vi "Scan1762testlongpulsetelegraph.vi"() -> ()   [LabVIEW 2012]
uses:
  <vilib>/DAQmx/write.llb/DAQmx Write (Digital Wfm 1Chan NSamp).vi
  <vilib>/DAQmx/create/channels.llb/DAQmx Create Channel (DO-Digital Output).vi
  <vilib>/DAQmx/configure/timing.llb/DAQmx Timing (Sample Clock).vi
  <vilib>/Waveform/DWDTOps.llb/DWDT Uncompress Digital.vi
  <vilib>/DAQmx/miscellaneous.llb/DAQmx Fill In Error Info.vi
  <vilib>/Utility/file.llb/Write To Spreadsheet File (DBL).vi
panel:
  out "10xwindow":i32
  out "10xdiscr":dbl
  out "DARK?":i32(graph)
  out "Counts":i32
  out "DARK?":bool
  out "PMT Counts":i32(graph)
  in  "PMT sample time":dbl=0.05
  out "Counts after 1762":i32=57
  out "OuterLoop":i32=101
  out "InnerLoop":i32=19
  out "Frequency Step Size":dbl=10000.0
  out "Bright Events":dbl
  in  "Discriminator Level\n (Bright/Dark)":i32=21
  out "number of samples written per channel\n(debug)":u32=42501
  out "digital waveform out 2":digitalwaveform(waveform)={"t0"=timestamp(0 s since 1904-01-01), "dt"=1e-07, "Y"={"transitions"=[0, 20000, 21001, 21501, 22501, 42500], "data"=[[1, 1, 0, 0], [0, 0, 0, 0], [0, 0, 0, 1], [0, 0, 0, 0], [1, 1, 0, 0], [1, 1, 0, 0]]}, "error"={"status"=FALSE, "code"=37421928, "source"=""}}
  in  "1762 pulse length (units of .1 us)":dbl=500.0
  in  "Comment":string="SPAOM, DPAOM = 77 MHz"
  in  "B Field":dbl=2.26
  in  "Power":dbl
  in  "Rerun BG Every\nnth freq point":dbl=20.0
  in  "PMT sample time":dbl=0.05
  out "Counts finding bright ion":dbl=39.0
  in  "BG Cutoff Limit":dbl=38.0
  in  "Runs per data point":dbl=20.0
  in  "Low Freq":dbl(slide)=81000000.0 min=50000000.0 max=120000000.0 step=1000.0 scale=75000000.0..90000000.0 scale format="%#.5f"
  in  "High Freq":dbl(slide)=86000000.0 min=50000000.0 max=120000000.0 step=1000.0 scale=80000000.0..90000000.0 scale format="%#.0f"
  out "Cur Freq":dbl=85984000.0 format="%#_8f"
  out "Path":path=path "c:/data/1762 Scans/2014-05-20_19-16-05_1762scanWithPumping.txt"
  out "Frequency Scan":cluster{dbl, dbl}[](graph)=[{87004000.0, 1.0}, {86994000.0, 1.0}, {86984000.0, 1.0}, {86974000.0, 1.0}, {86964000.0, 1.0}, {86954000.0, 1.0}, {86944000.0, 1.0}, {86934000.0, 1.0}, {86924000.0, 1.0}, {86914000.0, 1.0}, {86904000.0, 1.0}, {86894000.0, 1.0}, {86884000.0, 1.0}, {86874000.0, 1.0}, {86864000.0, 1.0}, {86854000.0, 1.0}, {86844000.0, 1.0}, {86834000.0, 1.0}, {86824000.0, 1.0}, {86814000.0, 1.0}, {86804000.0, 1.0}, {86794000.0, 1.0}, {86784000.0, 1.0}, {86774000.0, 1.0}, {86764000.0, 1.0}, {86754000.0, 1.0}, {86744000.0, 1.0}, {86734000.0, 1.0}, {86724000.0, 1.0}, {86714000.0, 1.0}, {86704000.0, 1.0}, {86694000.0, 1.0}, {86684000.0, 1.0}, {86674000.0, 1.0}, {86664000.0, 1.0}, {86654000.0, 1.0}, {86644000.0, 1.0}, {86634000.0, 1.0}, {86624000.0, 1.0}, {86614000.0, 1.0}, {86604000.0, 1.0}, {86594000.0, 1.0}, {86584000.0, 1.0}, {86574000.0, 1.0}, {86564000.0, 1.0}, {86554000.0, 1.0}, {86544000.0, 1.0}, {86534000.0, 1.0}, {86524000.0, 1.0}, {86514000.0, 1.0}, {86504000.0, 1.0}, {86494000.0, 1.0}, {86484000.0, 1.0}, {86474000.0, 1.0}, {86464000.0, 1.0}, {86454000.0, 1.0}, {86444000.0, 1.0}, {86434000.0, 1.0}, {86424000.0, 1.0}, {86414000.0, 1.0}, {86404000.0, 1.0}, {86394000.0, 1.0}, {86384000.0, 1.0}, {86374000.0, 1.0}, {86364000.0, 1.0}, {86354000.0, 1.0}, {86344000.0, 1.0}, {86334000.0, 1.0}, {86324000.0, 1.0}, {86314000.0, 1.0}, {86304000.0, 1.0}, {86294000.0, 1.0}, {86284000.0, 1.0}, {86274000.0, 1.0}, {86264000.0, 1.0}, {86254000.0, 1.0}, {86244000.0, 1.0}, {86234000.0, 1.0}, {86224000.0, 1.0}, {86214000.0, 1.0}, {86204000.0, 1.0}, {86194000.0, 1.0}, {86184000.0, 1.0}, {86174000.0, 1.0}, {86164000.0, 1.0}, {86154000.0, 1.0}, {86144000.0, 1.0}, {86134000.0, 1.0}, {86124000.0, 1.0}, {86114000.0, 1.0}, {86104000.0, 1.0}, {86094000.0, 1.0}, {86084000.0, 1.0}, {86074000.0, 1.0}, {86064000.0, 1.0}, {86054000.0, 1.0}, {86044000.0, 1.0}, {86034000.0, 1.0}, {86024000.0, 1.0}, {86014000.0, 1.0}, {86004000.0, 1.0}, {85994000.0, 1.0}]
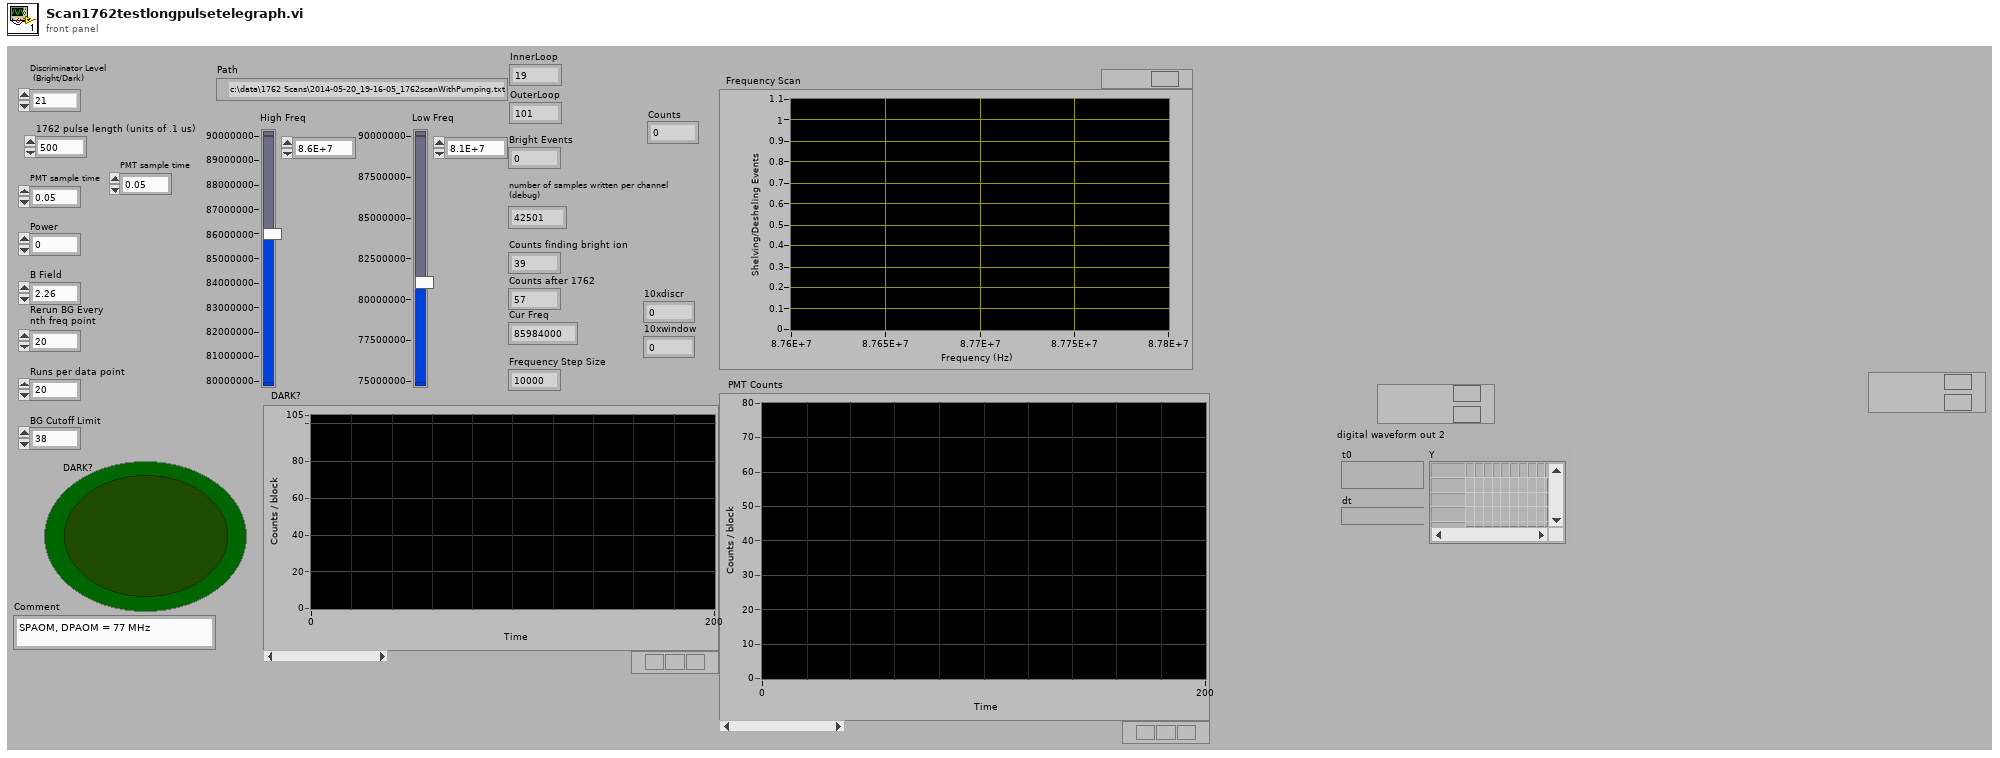
[diagram p1: front panel]
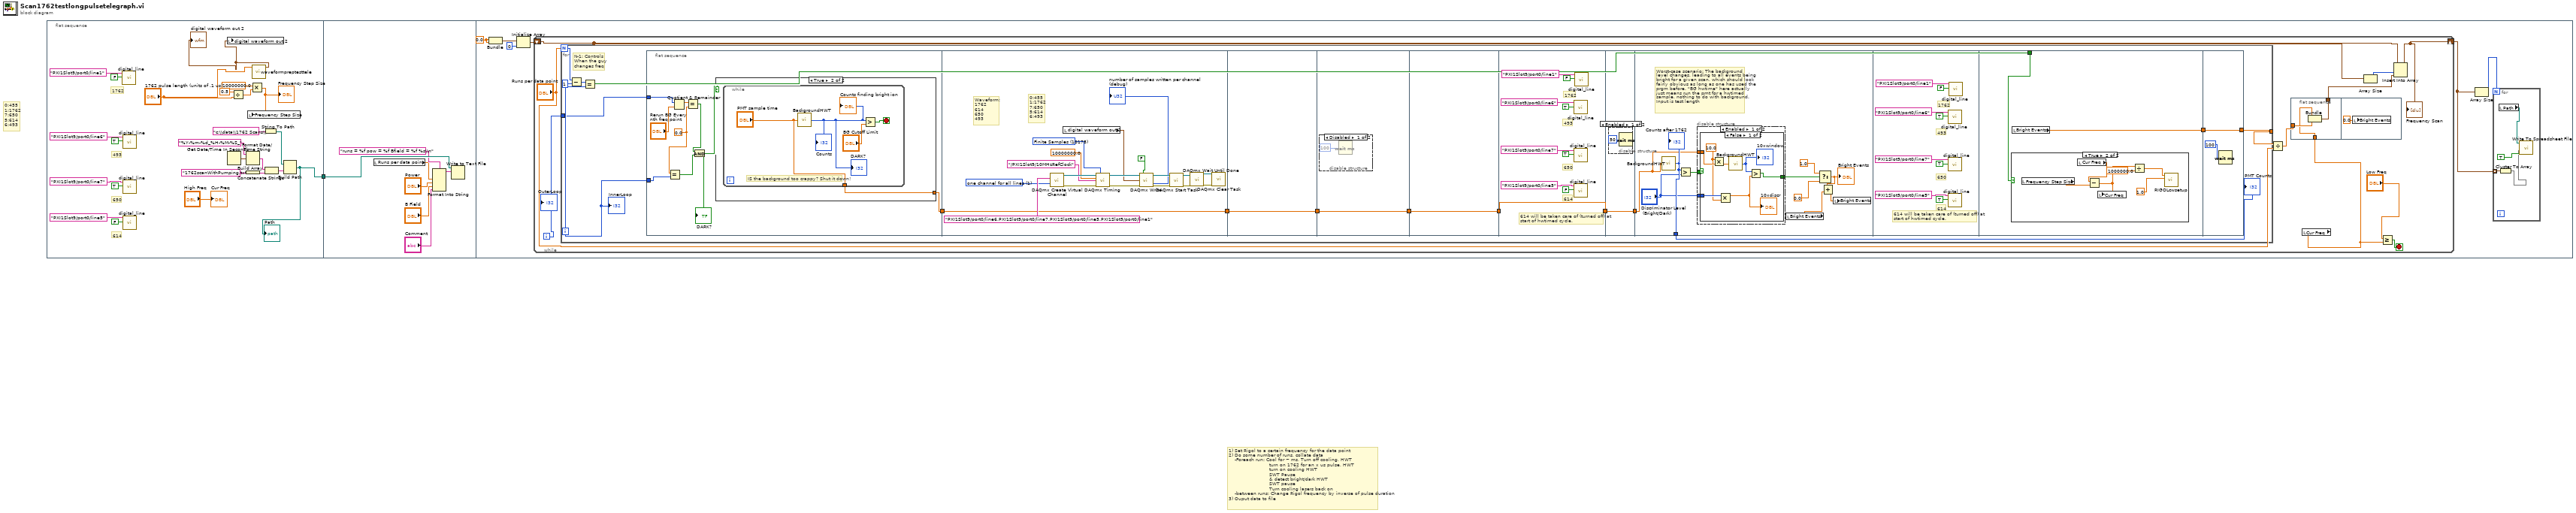
[diagram p0: block diagram]
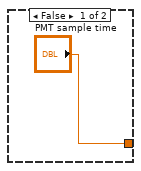
[diagram p2: hidden frame]
diagram:
  # "0:455\n1:1762\n7:650\n5:614\n6:493"
  # "1) Set Rigol to a certain frequency for the data point\n2) Do some number of runs, collate data\n    -Foreach run: Cool for ~ ms, Turn off cooling, HWT\n                           turn on 1762 for an x us pulse, HWT\n                           turn on cooling HWT\n                           SWT Pause\n                           & detect bright/dark HWT\n                           SWT pause\n                           Turn cooling lasers back on \n    -between runs: Change Rigol frequency by inverse of pulse duration\n3) Ouput data to file"
  n1 = flat-sequence {
    tunnel: [w17] -> w1
    tunnel: w1 -> [w32]
    frame #0 {
      # "614"
      # "650"
      # "493"
      # "1762"
      n2 = call "digital_line.vi"("Boolean"=FALSE, "lines"=tag "PXI1Slot9/port0/line1") -> ()  [unwired: 5 in, 1 out]
      n3 = call "digital_line.vi"("Boolean"=TRUE, "lines"=tag "PXI1Slot9/port0/line6") -> ()  [unwired: 5 in, 1 out]
      n4 = call "digital_line.vi"("Boolean"=TRUE, "lines"=tag "PXI1Slot9/port0/line7") -> ()  [unwired: 5 in, 1 out]
      n5 = call "digital_line.vi"("Boolean"=FALSE, "lines"=tag "PXI1Slot9/port0/line5") -> ()  [unwired: 5 in, 1 out]
      n6 = Get Date/Time In Seconds() -> (seconds since 1Jan1904=w19:timestamp)
      n7 = Divide(x=0.5, y="1762 pulse length (units of .1 us)") -> (x/y=w5:dbl)
      n8 = Format Date/Time String(time format string (%c)="%Y-%m-%d_%H-%M-%S_", seconds (now)=w19) -> (date/time string=w21:string)  [unwired: 1 in]
      n9 = Build Array("1762scanWithPumping.txt") -> (w24:string[])
      n10 = Multiply(x=10000000.0, y=w5) -> (x*y=w6:dbl)
      "Frequency Step Size" <- w6
      n11 = local write "Frequency Step Size"(w6) -> ()
      n12 = call "waveformpreptesttele.vi"("1762 pulse length (units of .1 us)"="1762 pulse length (units of .1 us)") -> ("digital waveform out 2"=w2:digitalwaveform)  [unwired: 8 in]
      "digital waveform out 2" <- w2
      n13 = local write "digital waveform out 2"(w2) -> ()
      n14 = String To Path(string="c:\\data\\1762 Scans\\") -> (path=w25:path)
      n15 = Concatenate Strings(w21, w24) -> (w23:string)
      n16 = Build Path(base path=w25, name or relative path=w23) -> (appended path=w17:path)
      "Path" <- w17
      "Cur Freq" <- "High Freq"
    }
    frame #1 {
      n17 = local read "Runs per data point"() -> (w29:dbl)
      n18 = Format Into String(format string="runs = %f pow = %f Bfield = %f %s\\n", w29, "Power", "B Field", "Comment") -> (resulting string=w30:string)  [unwired: 2 in, 1 out]
      n19 = Write to Text File(file (use dialog)=w32, text=w30) -> ()  [unwired: 2 in, 3 out]
    }
    frame #2 {
      w37 = 0.0
      n20 = Bundle(w37, w37) -> (w38:cluster{dbl, dbl})  [unwired: 1 in]
      n21 = Initialize Array(w38, 0) -> (w35:cluster{dbl, dbl}[])
      n22 = while {
        shift-right: [w49] -> w33
        shift-left: w35 -> [w50]
        i -> [w48]
        stop <- w52 stop-if-true
        n23 = for {
          N: "Runs per data point" -> [w70]
          tunnel: [w69] -> w45
          tunnel: w48 -> [w66]
          i -> [w67]
          # "N-1: Controls\nWhen the guy\nchanges freq"
          n24 = Subtract(x=w70, y=1) -> (x-y=w73:i32)
          n25 = Equal?(x=w73, y=w67) -> (x = y?=w71:bool)
          n26 = flat-sequence {
            tunnel: w67 -> [w80]
            tunnel: w66 -> [w75]
            tunnel: [w74] -> w65
            tunnel: [w90] -> w59
            tunnel: w65 -> [w90]
            tunnel: w59 -> [w108]
            tunnel: [w108] -> w58
            tunnel: w58 -> [w109]
            tunnel: [w109] -> w61
            tunnel: w61 -> [w111]
            tunnel: [w111] -> w60
            tunnel: w60 -> [w120]
            tunnel: [w120] -> w62
            tunnel: w62 -> [w121]
            tunnel: [w121] -> w63
            tunnel: w63 -> [w125]
            tunnel: [w127] -> w64
            tunnel: w71 -> [w154]
            tunnel: [w155] -> w68
            tunnel: [w163] -> w69
            tunnel: w68 -> [w163]
            frame #0 {
              w79 = 0.0 ("x")
              n27 = Equal?(x=w79, y=w80) -> (x = y?=w77:bool)
              n28 = Quotient & Remainder(x=w75, y="Rerun BG Every\nnth freq point") -> (x-y*floor(x/y)=w81:dbl)  [unwired: 1 out]
              n29 = Equal?(x=w81, y=w79) -> (x = y?=w78:bool)
              n30 = And(x=w78, y=w77) -> (x .and. y?=w76:bool)
              "DARK?" <- w76
              n31 = case shown="True" w76 {
                tunnel: ["PMT sample time" w84] -> w74
                frame False {
                }
                frame True {
                  n32 = while {
                    tunnel: ["PMT sample time"] -> w84
                    stop <- w87 stop-if-true
                    # "IS the background too crappy? Shut it down!"
                    n33 = call "BackgroundHWT.vi"("Sample Time(seconds)"="PMT sample time") -> ("Counts"=w85:i32)
                    "Counts finding bright ion" <- w85
                    "Counts" <- w85
                    "DARK?" <- w85
                    n34 = Greater?(x=w85, y="BG Cutoff Limit") -> (0:w87:bool)
                  }
                }
              }
            }
            frame #1 {
              w95 = 1 items=["one channel for each line", "one channel for all lines"] ("line grouping")
              w102 = 10178 items=["Finite Samples"=10178, "Continuous Samples"=10123, "Hardware Timed Single Point"=12522] ("sample mode")
              # "0:455\n1:1762\n7:650\n5:614\n6:493"
              # "Waveform:\n1762\n614\n650\n493"
              n35 = call-poly <vilib>:"DAQmx Create Virtual Channel.vi"("lines"=tag "PXI1Slot9/port0/line6,PXI1Slot9/port0/line7,PXI1Slot9/port0/line5,PXI1Slot9/port0/line1", "line grouping"=w95) -> ("task out"=w106:refnum<k21>, "error out"=w105:errorcluster)  [unwired: 12 in]
              n36 = local read "digital waveform out 2"() -> (w89:digitalwaveform)
              n37 = call-poly <vilib>:"DAQmx Timing.vi"("task/channels in"=w106, "sample mode"=w102, "rate"=10000000.0, "source"=tag "/PXI1Slot9/10MHzRefClock", "error in"=w105) -> ("task out"=w100:refnum<k21>, "error out"=w99:errorcluster)  [unwired: 9 in]
              n38 = call-poly <vilib>:"DAQmx Write.vi"("task/channels in"=w100, "auto start"=FALSE, "data"=w89, "error in"=w99) -> ("task out"=w98:refnum<k21>, "number of samples written per channel"=→"number of samples written per channel\n(debug)":u32, "error out"=w97:errorcluster)  [unwired: 9 in]
              n39 = call <vilib>:"DAQmx Start Task.vi"("task/channels in"=w98, "error in"=w97) -> ("task out"=w94:refnum<k21>, "error out"=w93:errorcluster)  [unwired: 12 in]
              n40 = call <vilib>:"DAQmx Wait Until Done.vi"("task/channels in"=w94, "error in"=w93) -> ("task out"=w91:refnum<k21>, "error out"=w92:errorcluster)  [unwired: 12 in]
              n41 = call <vilib>:"DAQmx Clear Task.vi"("task in"=w91, "error in"=w92) -> ()  [unwired: 13 in, 1 out]
            }
            frame #2 {
            }
            frame #3 {
              n42 = disable-structure shown="Disabled" {
                frame Disabled {
                  n43 = Wait (ms)(milliseconds to wait=u32 100) -> ()  [unwired: 1 out]
                }
                frame Enabled {
                }
              }
            }
            frame #4 {
            }
            frame #5 {
              # "614 will be taken care of (turned off) at\nstart of hwtimed cycle."
              # "614"
              # "650"
              # "493"
              # "1762"
              n44 = call "digital_line.vi"("Boolean"=TRUE, "lines"=tag "PXI1Slot9/port0/line6") -> ()  [unwired: 5 in, 1 out]
              n45 = call "digital_line.vi"("Boolean"=TRUE, "lines"=tag "PXI1Slot9/port0/line7") -> ()  [unwired: 5 in, 1 out]
              n46 = call "digital_line.vi"("Boolean"=FALSE, "lines"=tag "PXI1Slot9/port0/line5") -> ()  [unwired: 5 in, 1 out]
              n47 = call "digital_line.vi"("Boolean"=FALSE, "lines"=tag "PXI1Slot9/port0/line1") -> ()  [unwired: 5 in, 1 out]
            }
            frame #6 {
              n48 = disable-structure shown="Enabled" {
                frame Enabled {
                  n49 = Wait (ms)(milliseconds to wait=u32 50) -> ()  [unwired: 1 out]
                }
                frame Disabled {
                }
              }
            }
            frame #7 {
              # "Worst-case scenario: The background\nlevel changes, leading to all events being\nbright for a given scan, which should look\nfairly obvious as long as one has used the\nprgm before. \"BG hwtime\" here actually\njust means run the pmt for a hwtimed\nsample, nothing to do with background.\nInput is test length"
              n50 = call "BackgroundHWT.vi"("Sample Time(seconds)"=w125) -> ("Counts"=w127:i32)
              "Counts after 1762" <- w127
              n51 = Greater?(x=w127, y="Discriminator Level\n (Bright/Dark)") -> (0:w126:bool)
              n52 = disable-structure shown="Enabled" {
                disable-tunnel: w126 -> [w136 w145]
                disable-tunnel: [w135 w145] -> w123
                disable-tunnel: w125 -> [w134 _]
                disable-tunnel: "Discriminator Level\n (Bright/Dark)" -> [w133 _]
                frame Enabled {
                  n53 = case shown="False" w136 {
                    selector: w136 -> [_ w144]
                    tunnel: [w139 w144] -> w135
                    tunnel: w134 -> [w143 _]
                    tunnel: w133 -> [w140 _]
                    frame False {
                      w137 = 10.0 ("x")
                      n54 = Multiply(x=w137, y=w143) -> (x*y=w142:dbl)
                      n55 = Multiply(x=w140, y=w137) -> (x*y=w138:dbl)
                      "10xdiscr" <- w138
                      n56 = call "BackgroundHWT.vi"("Sample Time(seconds)"=w142) -> ("Counts"=w141:i32)
                      "10xwindow" <- w141
                      n57 = Greater?(x=w141, y=w138) -> (0:w139:bool)
                    }
                    frame True {
                    }
                  }
                }
                frame Disabled {
                }
              }
              n58 = local read "Bright Events"() -> (w128:dbl)
              n59 = Select(t=1.0, s=w123, f=0.0) -> (s? t:f=w130:dbl)
              "Bright Events" <- w130
              n60 = Add(x=w130, y=w128) -> (x+y=w129:dbl)
              n61 = local write "Bright Events"(w129) -> ()
            }
            frame #8 {
              # "614 will be taken care of (turned off) at\nstart of hwtimed cycle."
              # "614"
              # "650"
              # "493"
              # "1762"
              n62 = call "digital_line.vi"("Boolean"=TRUE, "lines"=tag "PXI1Slot9/port0/line6") -> ()  [unwired: 5 in, 1 out]
              n63 = call "digital_line.vi"("Boolean"=TRUE, "lines"=tag "PXI1Slot9/port0/line7") -> ()  [unwired: 5 in, 1 out]
              n64 = call "digital_line.vi"("Boolean"=TRUE, "lines"=tag "PXI1Slot9/port0/line5") -> ()  [unwired: 5 in, 1 out]
              n65 = call "digital_line.vi"("Boolean"=FALSE, "lines"=tag "PXI1Slot9/port0/line1") -> ()  [unwired: 5 in, 1 out]
            }
            frame #9 {
              n66 = case shown="True" w154 {
                frame False {
                }
                frame True {
                  n67 = local read "Frequency Step Size"() -> (w160:dbl)
                  n68 = local read "Cur Freq"() -> (w161:dbl)
                  n69 = Subtract(x=w161, y=w160) -> (x-y=w158:dbl)
                  n70 = local write "Cur Freq"(w158) -> ()
                  n71 = Divide(x=w158, y=1000000.0) -> (x/y=w156:dbl)
                  n72 = call "RIGOLcwsetup.vi"("Amplitude (Vpp)"=1.0, "Frequency (MHz)"=w156) -> ()  [unwired: 10 in]
                }
              }
              n73 = local read "Bright Events"() -> (w155:dbl)
            }
            frame #10 {
              n74 = Wait (ms)(milliseconds to wait=u32 100) -> ()  [unwired: 1 out]
            }
          }
          "InnerLoop" <- w67
          "PMT Counts" <- w64
        }
        n75 = Divide(x=w45, y="Runs per data point") -> (x/y=w44:dbl)
        n76 = flat-sequence {
          tunnel: w44 -> [w56]
          tunnel: [w55] -> w47
          tunnel: w46 -> [w54]
          frame #0 {
            n77 = Bundle("Cur Freq"=w54, w56) -> (w55:cluster{"Cur Freq":dbl, dbl})  [unwired: 1 in]
          }
          frame #1 {
            n78 = local write "Bright Events"(0.0 ("Bright Events")) -> ()
          }
        }
        n79 = local read "Cur Freq"() -> (w46:dbl)
        n80 = Array Size(array=w50) -> (size(s)=w51:i32)
        n81 = Greater Or Equal?(x="Low Freq", y=w46) -> (x >= y?=w52:bool)
        n82 = Insert Into Array(array=w50, index=w51, new element=w47) -> (w49:cluster{dbl, dbl}[])
        "Frequency Scan" <- w49
        "OuterLoop" <- w48
      }
      n83 = Array Size(array=w33) -> (size(s)=w34:i32)
      n84 = for {
        N: w34 -> [_]
        tunnel: w33 -> [w42] mode=indexing
        n85 = local read "Path"() -> (w39:path)
        n86 = Cluster To Array(cluster=w42) -> (array=w40:dbl[])
        n87 = call-poly <vilib>:"Write To Spreadsheet File.vi"("append to file? (new file:F)"=TRUE, "1D data"=w40, "file path (dialog if empty)"=w39) -> ()  [unwired: 5 in, 1 out]
      }
    }
  }
